vi "GetDigitalInputValues.vi"(8 "error in (no error)":errorcluster, 11 "wValues":i16) -> (0 "error out":errorcluster, 2 "function return":i16, 3 "wValues out":i16)   [LabVIEW 2013, in "HS3AcquireData.lvlib"]
doc: "Description: The TP112 has eight digital inputs, which are sampled simultaneously with the analog input channels.\nThis routine transfers the measured digital values from the memory in the DLL into the memory in the application. The measured data is returned in binary values. Each bit in the digital data words represents a digital input. wValues is an array. The caller must ensure that there is enough space in the array to contain the data. Therefore the size of the array in bytes must be at least RecordLength * sizeof(word)\nInput: -\nOutput: Return value E_NO_ERRORS | E_NOT_SUPPORTED | E_NO_HARDWARE\n\nFunction prototype: word GetDigitalInputValues( word *wValues )\n\nshort int GetDigitalInputValues ( short int *wValues );"
uses:
  HS3AcquireData.lvlib
  hs3.dll
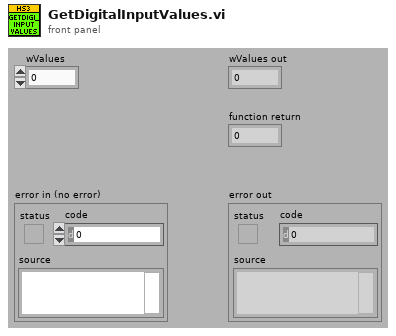
[diagram p1: front panel]
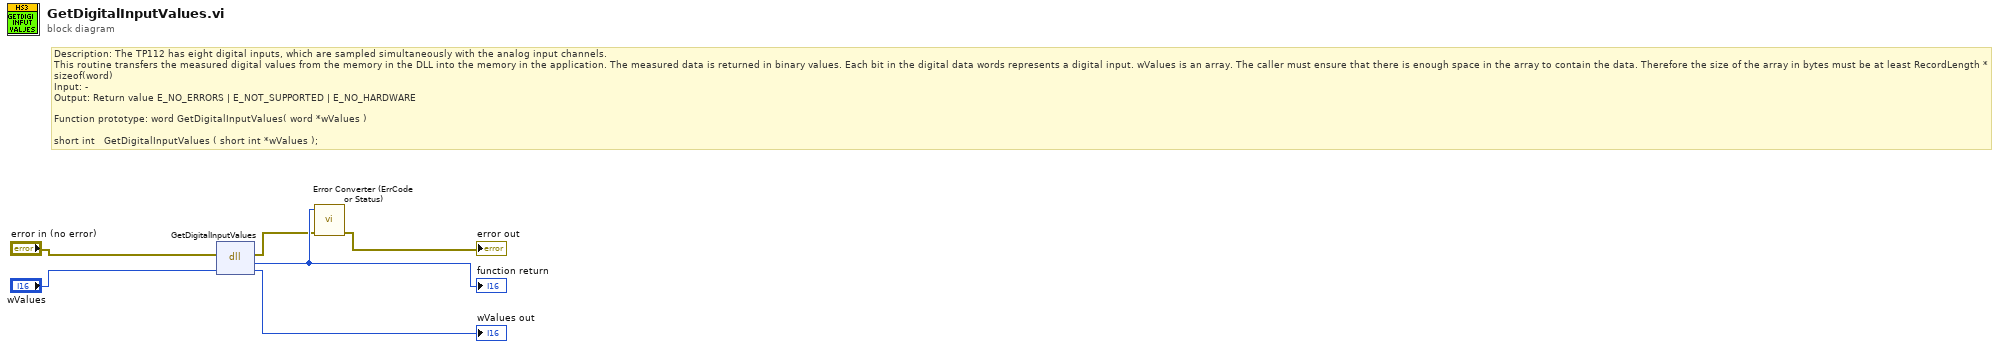
[diagram p0: block diagram]
diagram:
  # "Description: The TP112 has eight digital inputs, which are sampled simultaneously with the analog input channels.\nThis routine transfers the measured digital values from the memory in the DLL into the memory in the application. The measured data is returned in binary values. Each bit in the digital data words represents a digital input. wValues is an array. The caller must ensure that there is enough space in the array to contain the data. Therefore the size of the array in bytes must be at least RecordLength * sizeof(word)\nInput: -\nOutput: Return value E_NO_ERRORS | E_NOT_SUPPORTED | E_NO_HARDWARE\n\nFunction prototype: word GetDigitalInputValues( word *wValues )\n\nshort int \t\tGetDigitalInputValues\t( short int *wValues );"
  n1 = dll-call lib="C:/Documents and Settings/admin/Pulpit/HS3 LabViewLib/HS3_WRAPPER/AcquireData/hs3.*" fn="GetDigitalInputValues"(error in="error in (no error)", "wValues"="wValues") -> (error out=w2:errorcluster, w6:i16, "wValues"=→"wValues out":i16)  [unwired: 2 in, 1 out]
  "function return" <- w6
  n2 = call "Error Converter (ErrCode or Status).vi"("error in (no error)"=w2, "error code"=w6) -> ("error out"=→"error out":errorcluster)  [unwired: 9 in]
